vi "rqcBob Configure PD State FIFO.vi"(8 "error in":errorcluster, 9 "PD.state fifo depth":u32=1000000, 10 "PD.state fifo write enable":bool, 11 "FPGA reference in":refnum<k20>) -> (0 "error out":errorcluster, 3 "FPGA reference out":refnum<k20>)   [LabVIEW 2018]
uses:
  <vilib>/Utility/error.llb/Error Cluster From Error Code.vi
  <vilib>/rvi/errors/niLvFpgaAdjustHostInterfaceError.vi
  <vilib>/rvi/interface/common/niFpgaWaitOnOcc.vi
  <vilib>/rvi/interface/nirviReadWriteControl/nirviReadWriteControl.xnode
  <vilib>/rvi/interface/nirviMethod/nirviMethod.xnode
  <vilib>/rvi/errors/niLvFpgaMergeErrorWithErrorCode.vi
  NiFpgaLv.dll
  <vilib>/rvi/interface/Simulation/niFpgaSimulationCallBeginRW.vi
  <vilib>/FPGAPlugInAG/Dynamic/niLvFpga_ConfigureFifo_Dynamic.vi
  <vilib>/FPGAPlugInAG/Dynamic/niLvFpga_StartFifo_Dynamic.vi
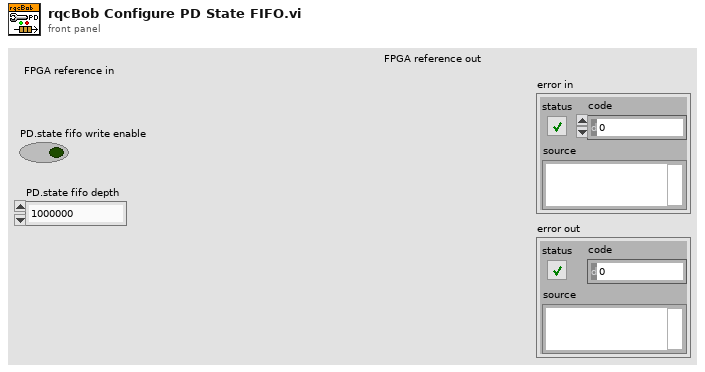
[diagram p1: front panel]
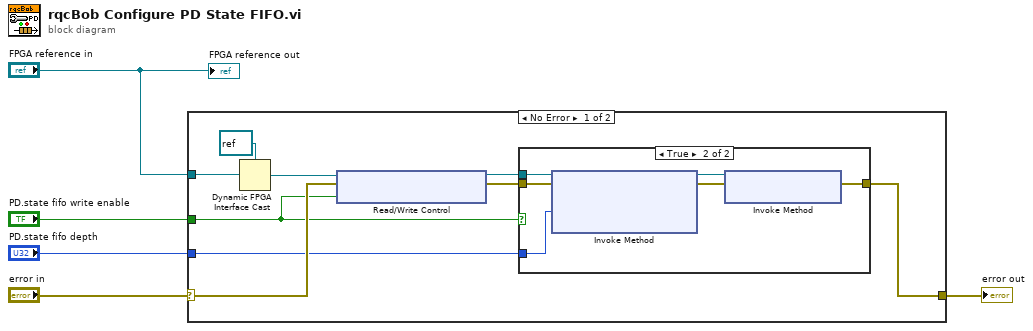
[diagram p0: block diagram]
diagram:
  n1 = case shown="No Error" "error in" {
    selector: "error in" -> [w14 w22]
    tunnel: [w8 w22] -> w3
    tunnel: "FPGA reference in" -> [w12 _]
    tunnel: "PD.state fifo write enable" -> [w6 _]
    tunnel: "PD.state fifo depth" -> [w7 _]
    frame No Error {
      n2 = Dynamic FPGA Interface Cast(Session In=refnum<k20> refnum ("FPGA Interface"), Type=w12) -> (Session Out=w11:refnum<k20>)
      n3 = xnode "Read/Write Control"("FPGA VI Reference In"=w11, "error in"=w14, "PD.state fifo write enable"=w6) -> ("FPGA VI Reference Out"=w10:refnum<k20>, "error out"=w9:errorcluster)
      n4 = case shown="True" w6 {
        tunnel: w10 -> [_ w21]
        tunnel: w9 -> [w15 w20]
        tunnel: [w15 w16] -> w8
        tunnel: w7 -> [_ w19]
        frame False {
        }
        frame True {
          n5 = xnode "Invoke Method"("FPGA VI Reference In"=w21, "error in"=w20, "Requested Depth"=w19) -> ("FPGA VI Reference Out"=w18:refnum<k20>, "error out"=w17:errorcluster)  [unwired: 1 out]
          n6 = xnode "Invoke Method"("FPGA VI Reference In"=w18, "error in"=w17) -> ("error out"=w16:errorcluster)  [unwired: 1 out]
        }
      }
    }
    frame Error {
    }
  }
  "error out" <- w3
  "FPGA reference out" <- "FPGA reference in"
